vi "_FPGA Runtime Update.vi"(4 "error in":errorcluster, 6 "Parameters":T1[](array[typedef])) -> (0 "error out":errorcluster)   [LabVIEW 2012]
uses:
  Type/_RT Active Ch.ctl
  _RT Global.vi
  <vilib>/Utility/error.llb/Error Cluster From Error Code.vi
  <vilib>/rvi/errors/niLvFpgaAdjustHostInterfaceError.vi
  <vilib>/rvi/interface/nirviReadWriteControl/nirviReadWriteControl.xnode
  FPGA Bitfiles/FPGA9602.lvbitx
  NiFpgaLv.dll
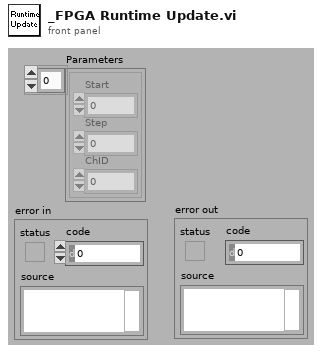
[diagram p1: front panel]
types:
  T1 = typedef "_RT Active Ch.ctl" = cluster{"Start":i32, "Step":i32, "ChID":i32}
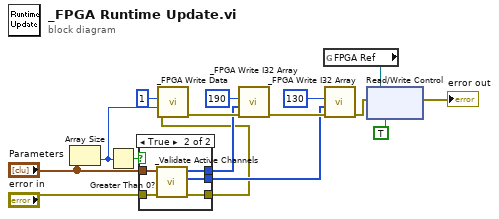
[diagram p0: block diagram]
diagram:
  n1 = Array Size(array="Parameters") -> (size(s)=w5:i32)
  n2 = Greater Than 0?(x=w5) -> (x > 0?=w7:bool)
  n3 = case shown="True" w7 {
    tunnel: [w17 w22] -> w2
    tunnel: "Parameters" -> [_ w21]
    tunnel: [_ w20] -> w4
    tunnel: [_ w19] -> w3
    tunnel: "error in" -> [w17 w18]
    frame False {
    }
    frame True {
      n4 = call "_Validate Active Channels.vi"("error in"=w18, "Active Ch"=w21) -> ("error out"=w22:errorcluster, "DAC Values"=w19:i32[], "Ch ID"=w20:i32[])  [unwired: 4 in, 1 out]
    }
  }
  n5 = call "_FPGA Write Data.vi"("error in"=w2, "Data"=w5, "Address"=u16 1) -> ("error out"=w16:errorcluster)  [unwired: 3 in, 2 out]
  n6 = call "_FPGA Write I32 Array.vi"("error in"=w16, "I32 Array"=w4, "Offset (0)"=u16 190 ("Address")) -> ("error out"=w10:errorcluster)  [unwired: 2 in, 2 out]
  n7 = global read "_RT Global.vi" "FPGA Ref"() -> (w1:refnum<k20>)
  n8 = call "_FPGA Write I32 Array.vi"("error in"=w10, "I32 Array"=w3, "Offset (0)"=u16 130 ("Address")) -> ("error out"=w13:errorcluster)  [unwired: 2 in, 2 out]
  n9 = xnode "Read/Write Control"("FPGA VI Reference In"=w1, "error in"=w13, "Update"=TRUE ("Start")) -> ("error out"=→"error out":errorcluster)  [unwired: 1 out]
